vi "Remove Empty Properties.vi"(10 "Values in":string[](array[string]), 11 "Names in":string[](array[string])) -> (2 "Values out":string[](array[string]), 3 "Names out":string[](array[string]))   [LabVIEW 2017, in "LabVIEW CycloneDX SBOM.lvlib" / "CycloneDX JSON.lvclass"]
doc: "Remove properties (names) where the value is an empty string or '0'."
uses:
  CycloneDX JSON.lvclass
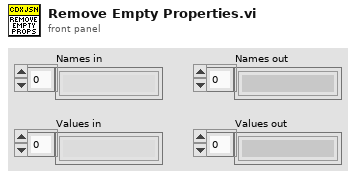
[diagram p1: front panel]
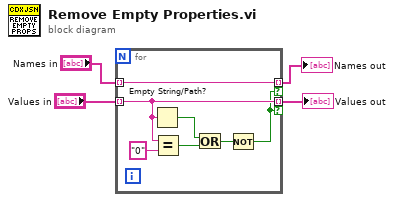
[diagram p0: block diagram]
diagram:
  n1 = for {
    tunnel: "Values in" -> [w7] mode=indexing
    tunnel: "Names in" -> [w8] mode=indexing
    tunnel: [w8] -> w3 mode=indexing if=w5
    tunnel: [w7] -> w4 mode=indexing if=w5
    n2 = Empty String/Path?(string/path=w7) -> (empty?=w10:bool)
    n3 = Equal?(x=w7, y="0") -> (x = y?=w11:bool)
    n4 = Or(x=w10, y=w11) -> (x .or. y?=w6:bool)
    n5 = Not(x=w6) -> (.not. x?=w5:bool)
  }
  "Values out" <- w4
  "Names out" <- w3
